vi "pf_Extract_Ports_Info.vi"(8 "error in (no error)":errorcluster, 10 "Ports Array":string[](array[string])=["0, National Instruments, img0::0, 3, 0", "1, RS-232, com1, 0, 3", "2, RS-232, com2, 0, 3", "3, RS-232, com3, 0, 3", "4, RS-232, com4, 0, 3"]) -> (0 "error out":errorcluster, 2 "Ports Info Array":T1[](array[typedef]))   [LabVIEW 2025, in "Photonfocus_Toolkit.lvlib"]
uses:
  Photonfocus_Toolkit.lvlib
  _Private/Controls/pf_Port_Info.ctl
  _Private/Controls/pf_CLALLSERIAL_Version.ctl
  _Private/Controls/pf_Port_Type.ctl
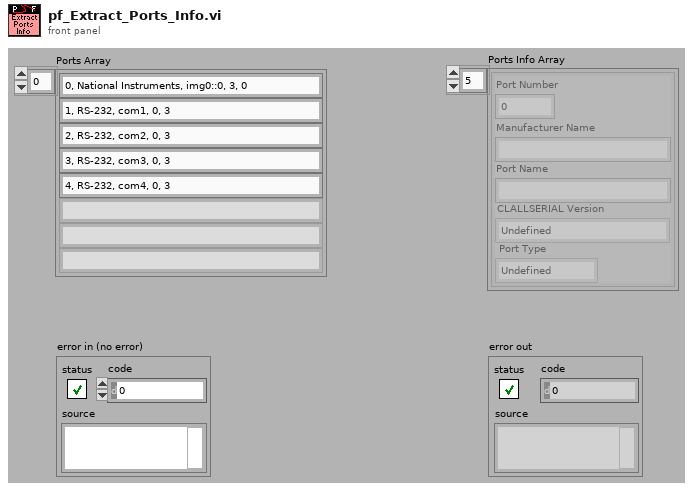
[diagram p1: front panel]
types:
  T1 = typedef "Photonfocus_Toolkit.lvlib/pf_Port_Info.ctl" = cluster{"Port Number":i32, "Manufacturer Name":string, "Port Name":string, "CLALLSERIAL Version":T2, "Port Type":T3}
  T2 = typedef "Photonfocus_Toolkit.lvlib/pf_CLALLSERIAL_Version.ctl" = enum16{"Undefined", "No CLALLSERIAL port", "CL_DLL_VERSION_NO_VERSION", "CL_DLL_VERSION_1_0", "CL_DLL_VERSION_1_1"}
  T3 = typedef "Photonfocus_Toolkit.lvlib/pf_Port_Type.ctl" = enum16{"Undefined", "CLALLSERIAL port", "port with clser.dll", "USB port", "RS-232 port"}
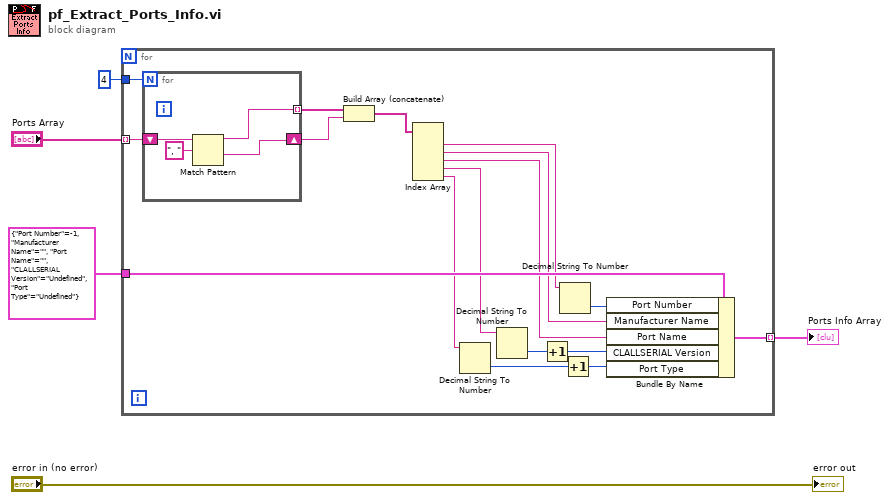
[diagram p0: block diagram]
diagram:
  n1 = for {
    tunnel: "Ports Array" -> [w22] mode=indexing
    tunnel: 4 -> [w21]
    tunnel: T1 {"Port Number"=-1, "Manufacturer Name"="", "Port Name"="", "CLALLSERIAL Version"=enum."Undefined", "Port Type"=enum."Undefined"} ("Port Info") -> [w20]
    tunnel: [w14] -> w2 mode=indexing
    n2 = for {
      N: w21 -> [_]
      shift-right: [w24] -> w9
      shift-left: w22 -> [w26]
      tunnel: [w23] -> w7 mode=indexing
      n3 = Match Pattern(string=w26, regular expression=", ") -> (before substring=w23:string, after substring=w24:string)  [unwired: 3 out]
    }
    n4 = Build Array (concatenate)(w7, w9) -> (w8:string[])
    n5 = Index Array(array=w8) -> (element #1=w15:string, element #2=w19:string, element #3=w6:string, element #4=w18:string, element #5=w17:string)  [unwired: 5 in]
    n6 = Decimal String To Number(string=w17) -> (number=w11:i32)  [unwired: 3 out]
    n7 = Decimal String To Number(string=w18) -> (number=w13:i32)  [unwired: 3 out]
    n8 = Increment(x=w13) -> (x+1=w12:i32)
    n9 = Decimal String To Number(string=w15) -> (number=w16:i32)  [unwired: 3 out]
    n10 = Increment(x=w11) -> (x+1=w10:i32)
    n11 = Bundle By Name(cluster=w20, "Port Number"=w16, "Manufacturer Name"=w19, "Port Name"=w6, "CLALLSERIAL Version"=w12, "Port Type"=w10) -> (w14:T1)
  }
  "Ports Info Array" <- w2
  "error out" <- "error in (no error)"
